vi "HRM-Hardware_main.vi"(8 "error in (no error)":errorcluster, 11 "Init cluster":T1) -> (0 "error out":errorcluster)   [LabVIEW 2020]
uses:
  HRM-init_cluster.ctl
  HRM-User_events.ctl
panel:
  in  "stop":bool
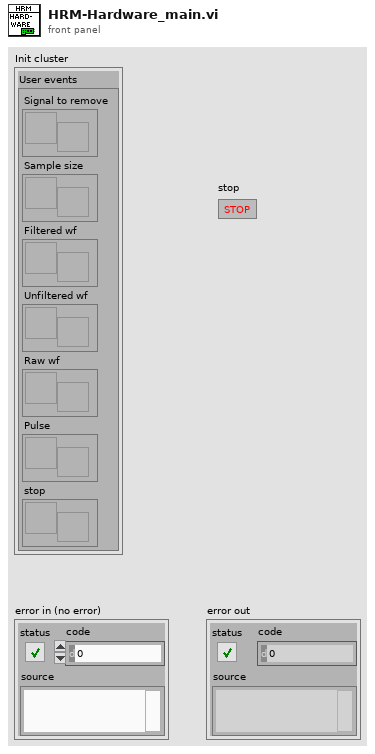
[diagram p1: front panel]
types:
  T1 = typedef "HRM-init_cluster.ctl" = cluster{"User events":T2}
  T2 = typedef "HRM-User_events.ctl" = cluster{"Signal to remove":refnum<user-event>, "Sample size":refnum<user-event>, "Filtered wf":refnum<user-event>, "Unfiltered wf":refnum<user-event>, "Raw wf":refnum<user-event>, "Pulse":refnum<user-event>, "stop":refnum<user-event>}
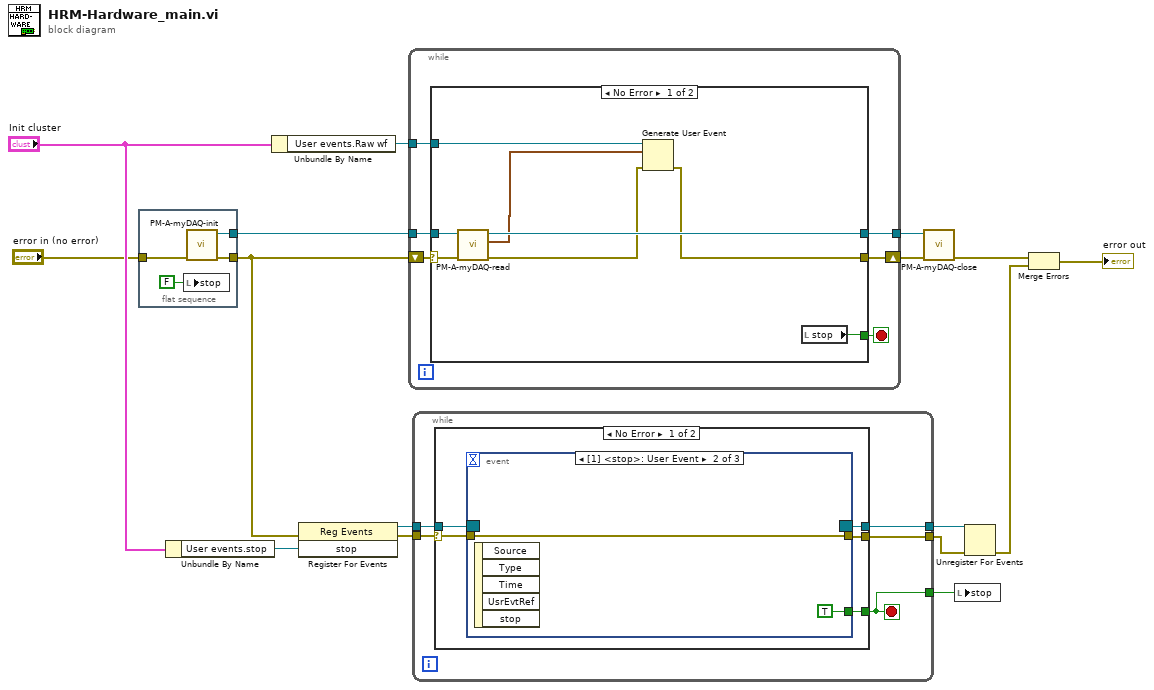
[diagram p0: block diagram]
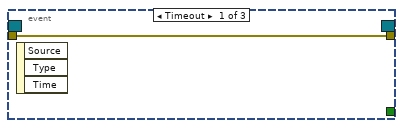
[diagram p2: hidden frame]
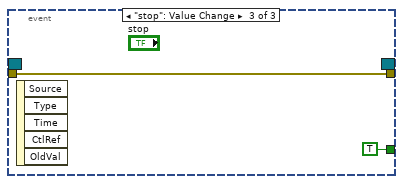
[diagram p3: hidden frame]
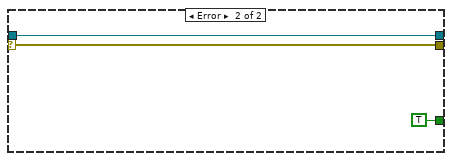
[diagram p4: hidden frame]
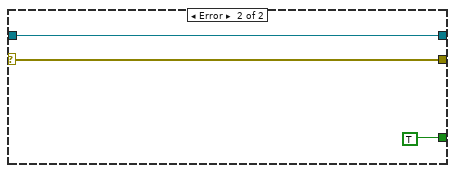
[diagram p5: hidden frame]
diagram:
  n1 = flat-sequence {
    tunnel: "error in (no error)" -> [w20]
    tunnel: [w19] -> w5
    tunnel: [w17] -> w2
    frame #0 {
      n2 = local write "stop"(FALSE ("stop")) -> ()
      n3 = call "PM-A-myDAQ-init.vi"("error in"=w20) -> ("error out"=w17:errorcluster, "Refnum out"=w19:refnum<k21>)  [unwired: 9 in]
    }
  }
  n4 = Unbundle By Name("Init cluster") -> ("User events.stop"=w8:refnum<user-event>)
  n5 = Unbundle By Name("Init cluster") -> ("User events.Raw wf"=w6:refnum<user-event>)
  n6 = register-events(error in=w2, w8) -> (reference out=w11:refnum<event-registration>, error out=w7:errorcluster)  [unwired: 1 in]
  n7 = while {
    tunnel: w5 -> [w26]
    tunnel: [w24] -> w4
    shift-right: [w23] -> w3
    shift-left: w2 -> [w25]
    tunnel: w6 -> [w21]
    stop <- w22 stop-if-true
    n8 = case shown="No Error" w25 {
      selector: w25 -> [w33 w36]
      tunnel: w26 -> [w34 w35]
      tunnel: [w32 w35] -> w24
      tunnel: [w29 w36] -> w23
      tunnel: [w27 TRUE ("Stop")] -> w22
      tunnel: w21 -> [w28 _]
      frame No Error {
        n9 = call "PM-A-myDAQ-read.vi"("error in (no error)"=w33, "Refnum in"=w34) -> ("error out"=w30:errorcluster, "data"=w31:waveform(dbl), "Refnum out"=w32:refnum<k21>)  [unwired: 7 in]
        n10 = Generate User Event(user event=w28, event data cluster=w31, error in=w30) -> (error out=w29:errorcluster)  [unwired: 1 in, 1 out]
        n11 = local read "stop"() -> (w27:bool)
      }
      frame Error {
      }
    }
  }
  n12 = while {
    tunnel: w7 -> [w42]
    tunnel: w11 -> [w41]
    tunnel: [w40] -> w12
    tunnel: [w39] -> w13
    tunnel: [w38] -> w1
    stop <- w38 stop-if-true
    n13 = case shown="No Error" w42 {
      selector: w42 -> [w45 w54]
      tunnel: w41 -> [w47 w53]
      tunnel: [w46 TRUE] -> w38
      tunnel: [w44 w54] -> w39
      tunnel: [w43 w53] -> w40
      frame No Error {
        n14 = event shown="[1] <stop>: User Event" {
          selector: w47 -> [_ _ _]
          dyn-events: [_ _ _] -> w43
          timeout: _ -> [_ _ _]
          tunnel: [_ TRUE TRUE] -> w46
          tunnel: w45 -> [w48 w49 w52]
          tunnel: [w48 w49 w52] -> w44
          event Timeout {
            n15 = event-data() -> ()  [unwired: 1 in, 3 out]
          }
          event User Event {
            n16 = event-data() -> ()  [unwired: 1 in, 5 out]
          }
          event "stop": Value Change {
            n17 = event-data() -> ()  [unwired: 1 in, 5 out]
          }
        }
      }
      frame Error {
      }
    }
  }
  n18 = call "PM-A-myDAQ-close.vi"("error in (no error)"=w3, "Refnum in"=w4) -> ("error out"=w14:errorcluster)  [unwired: 9 in]
  n19 = local write "stop"(w1) -> ()
  n20 = Unregister For Events(event registration refnum=w12, error in=w13) -> (error out=w15:errorcluster)
  n21 = Merge Errors(w14, w15) -> (→"error out":errorcluster)
